vi "Field.vi"(4 "channel 2":T2, 6 "Draw Targets?":T1, 7 "AutoScale":bool=TRUE, 8 "channel for IA State":T3, 10 "Scale mm/pixel":dbl=1.0 format="%#_13g", 11 "channel":T4) -> (2 "Scale Out":dbl, 3 "2D Picture":picture, 5 "AutoScale Out":bool=TRUE)   [LabVIEW 2017]
uses:
  <vilib>/Utility/miscctls.llb/LVBoundsTypeDef.ctl
  <extravilib>/ChannelInstances/Lossy Stream-t'AI Input.ctl'.lvlib
  <extravilib>/ChannelInstances/Lossy Stream-a[.](i32).lvlib
  <extravilib>/ChannelInstances/Lossy Stream-t'SSL Field State.ctl'.lvlib
  Intel/Functions Enum.ctl
  Core/AI Robot.ctl
  Core/AI Ball.ctl
  Core/Field Size.ctl
  Intel/Command Enum.ctl
  Core/AI Judge.ctl
  Core/AI Input.ctl
  <extravilib>/ChannelInstances/Lossy Stream-t'AI Input.ctl'/)Channel.ctl
  <vilib>/Analysis/Matrix/Datatypes/RealMatrix.ctl
  <vilib>/Analysis/Matrix/NI_Matrix.lvlib
  SSL Detection Robot.ctl
  SSL Detection Ball.ctl
  SSL Detection Frame.ctl
  SSL/SSL Field State.ctl
  <extravilib>/ChannelInstances/Lossy Stream-t'SSL Field State.ctl'/)Channel.ctl
  <extravilib>/ChannelInstances/Lossy Stream-a[.](i32)/)Channel.ctl
  Intel/AttackerStates.ctl
  Util/Events/Events.ctl
  DrawTargets.ctl
panel:
  in  "Draw Number":bool=TRUE
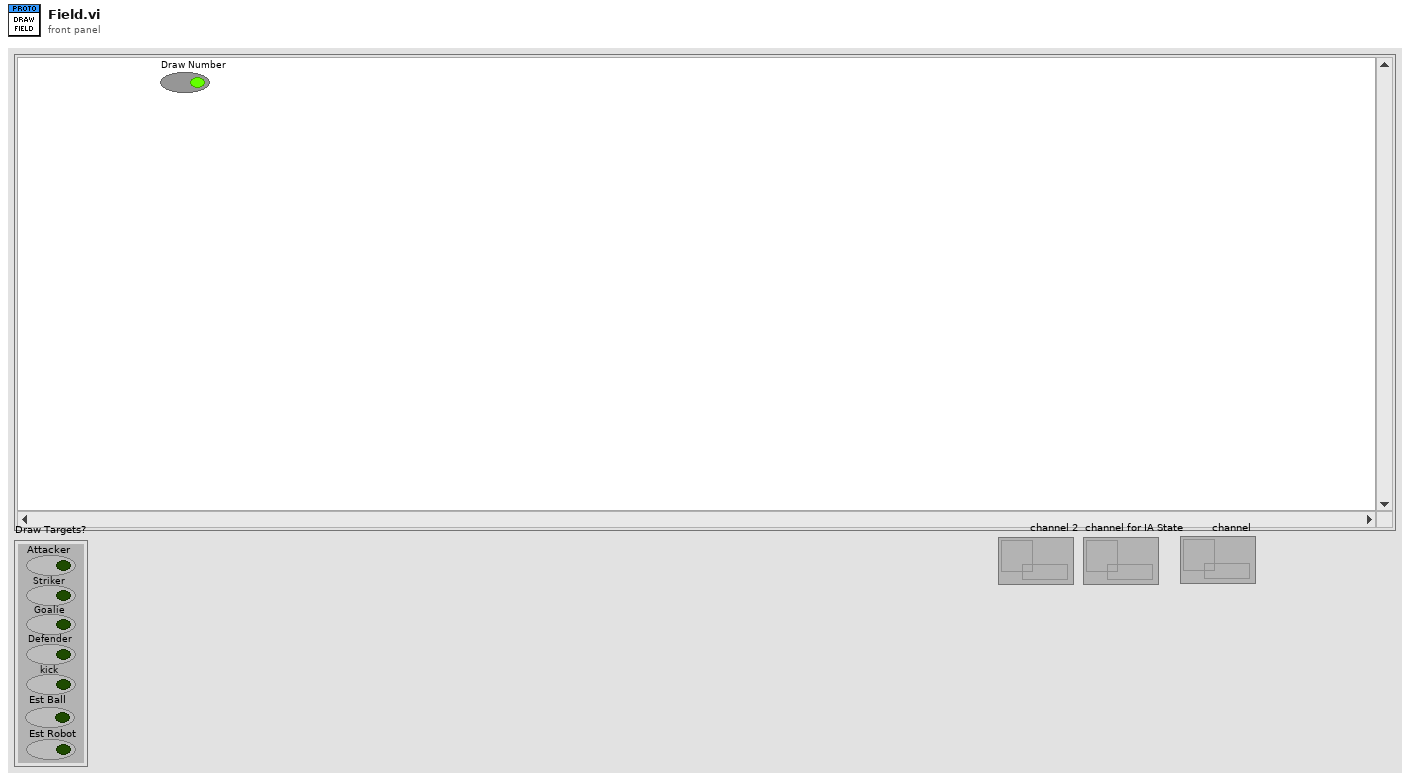
[diagram p1: front panel]
types:
  T1 = typedef "DrawTargets.ctl" = cluster{"Attacker":bool, "Striker":bool, "Goalie":bool, "Defender":bool, "kick":bool, "Est Ball":bool, "Est Robot":bool}
  T2 = typedef "Lossy Stream-a[.](i32).lvlib/)Channel.ctl" = refnum<queue>
  T3 = typedef "Lossy Stream-t'AI Input.ctl'.lvlib/)Channel.ctl" = refnum<queue>
  T4 = typedef "Lossy Stream-t'SSL Field State.ctl'.lvlib/)Channel.ctl" = refnum<queue>
  T5 = typedef "LVBoundsTypeDef.ctl" = cluster{"Width":u32, "Height":u32}
  T6 = typedef "SSL Field State.ctl" = cluster{"Detection Frame Out":T7, "Field Size Out":cluster{"line_width":u32, "field_length":u32, "field_width":u32, "boundary_width":u32, "referee_width":u32, "goal_width":u32, "goal_depth":u32, "goal_wall_width":u32, "center_circle_radius":u32, "defense_radius":u32, "defense_stretch":u32, "free_kick_from_defense_dist":u32, "penalty_spot_from_field_line_dist":u32, "penalty_line_from_spot_dist":u32}, "Received Time Stamp":timestamp}
  T7 = typedef "SSL Detection Frame.ctl" = cluster{"frame_number":u32, "t_capture":dbl, "t_sent":dbl, "camera_id":u32, "robots_yellow":T8[], "robots_blue":T8[], "balls":T10[], "Valid":bool, "Time Stamp":timestamp}
  T8 = typedef "SSL Detection Robot.ctl" = cluster{"x":sgl, "robot_id":u32, "confidence":sgl, "y":sgl, "orientation":sgl, "pixel_x":sgl, "pixel_y":sgl, "height":sgl, "Valid":bool, "Time Stamp":timestamp, "x_k|k":T9, "Pk|k":T9, "Previous Time Stamp":timestamp, "R":T9}
  T9 = typedef "NI_Matrix.lvlib/RealMatrix.ctl" = dbl[][]
  T10 = typedef "SSL Detection Ball.ctl" = cluster{"x":sgl, "area":u32, "confidence":sgl, "y":sgl, "z":sgl, "pixel_x":sgl, "pixel_y":sgl, "Valid":bool, "Time Stamp":timestamp, "x_k|k":T9, "Pk|k":T9, "Id":u32, "Previous Time Stamp":timestamp, "R":T9}
  T11 = typedef "AI Input.ctl" = cluster{"our_robots":T12[], "enemy_robots":T12[], "balls":T15[], "geometry":T16, "IA Judge":T17, "Received Timestamp":timestamp, "Events":T19}
  T12 = typedef "AI Robot.ctl" = cluster{"id":u32, "function":T13, "x":dbl, "y":dbl, "orientation":dbl, "v_tangent":dbl, "v_normal":dbl, "v_ang":dbl, "kick_x":dbl, "kick_z":dbl, "dribble":bool, "Timestamp":timestamp, "dest_x":dbl, "dest_y":dbl, "dest_orientation":dbl, "estimatives":cluster{"est_v_tangent":dbl, "est_v_normal":dbl, "est_vx":dbl, "est_vy":dbl, "Pos Robot Est":dbl[]}, "dest_x_kick":dbl, "dest_y_kick":dbl, "Gap Coord":dbl[], "States":T14}
  T13 = typedef "Functions Enum.ctl" = enum16{"Attacker", "Goalie", "Defender", "Striker", "Goto 0", "Dummy", "Kicker", "ZigZag"}
  T14 = typedef "AttackerStates.ctl" = enum16{"Pass", "GoToTangent", "BallGetting", "GoToKick", ""}
  T15 = typedef "AI Ball.ctl" = cluster{"x":dbl, "y":dbl, "timestamp":timestamp, "Vel_x":dbl, "Vel_y":dbl, "Pos Bola Est":dbl[]}
  T16 = typedef "Field Size.ctl" = cluster{"line_width":u32, "field_length":u32, "field_width":u32, "boundary_width":u32, "referee_width":u32, "goal_width":u32, "goal_depth":u32, "goal_wall_width":u32, "center_circle_radius":u32, "defense_radius":u32, "defense_stretch":u32, "free_kick_from_defense_dist":u32, "penalty_spot_from_field_line_dist":u32, "penalty_line_from_spot_dist":u32}
  T17 = typedef "AI Judge.ctl" = cluster{"stage":string, "command":string, "our_goalie_id":dbl, "enemy_goalie_id":dbl, "command enum":T18, "Time":enum16{"Azul", "Amarelo"}}
  T18 = typedef "Command Enum.ctl" = enum16{"Halt", "Stop", "Force Start", "PKA Normal Start", "Prepare Kickoff Ally", "PKE Normal Start", "Prepare Kickoff Enemy", "Prepare Penalty Ally", "PPA Normal Start", "Prepare Penalty Enemy", "PPE Normal Start", "Direct Free Enemy", "Direct Free Ally", "Indirect Free Enemy", "Indirect Free Ally", "Timeout Enemy", "Timeout Ally", "Goal Enemy", "Goal Ally", "Ball Placement Enemy", "Ball Placement Ally", "Normal Half Time", "Extra Time Break", "Extra Half Time", "None", "Post Game"}
  T19 = typedef "Events.ctl" = cluster{"Touch":bool, "Ball out":bool, "id touch":dbl, "Ball out of \nVision":bool, "Ball inside \nGoalie area":bool, "Robot not responding":bool, "Robots responding status":dbl[], "Enemy Ball \nPossession":bool, "Pass State":bool, "id end of pass":dbl, "Kick":bool, "Id ini Possession":dbl, "Ball Possesion":bool, "Id Possesion":dbl}
  T20 = cluster{"line_width":u32, "field_length":u32, "field_width":u32, "boundary_width":u32, "referee_width":u32, "goal_width":u32, "goal_depth":u32, "goal_wall_width":u32, "center_circle_radius":u32, "defense_radius":u32, "defense_stretch":u32, "free_kick_from_defense_dist":u32, "penalty_spot_from_field_line_dist":u32, "penalty_line_from_spot_dist":u32}
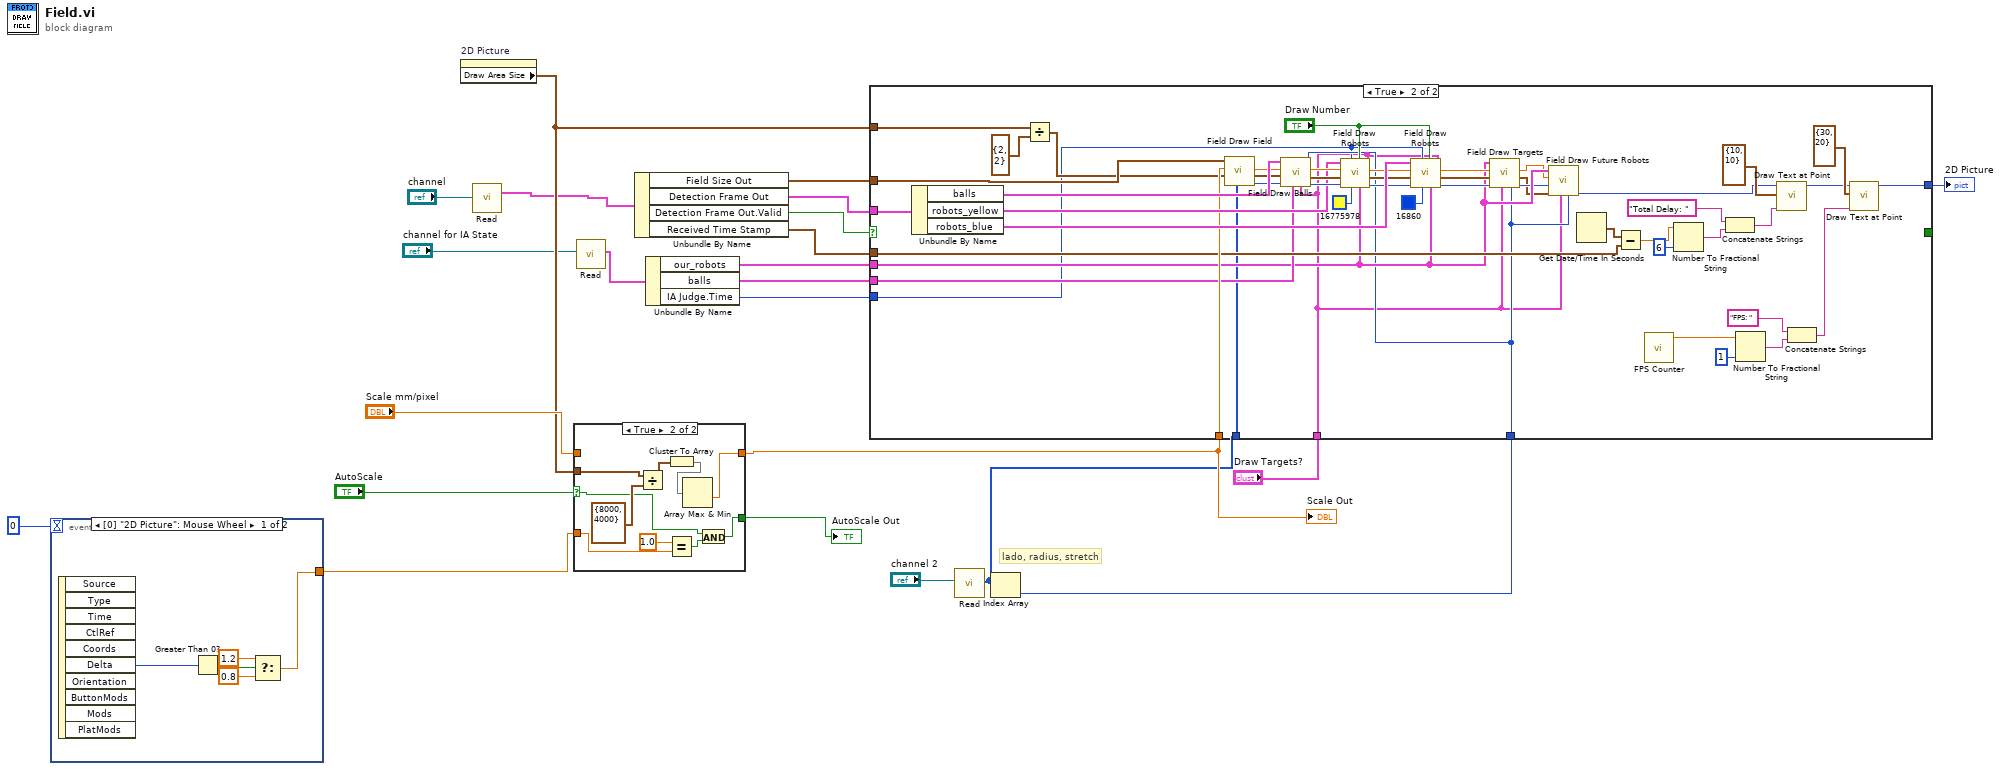
[diagram p0: block diagram]
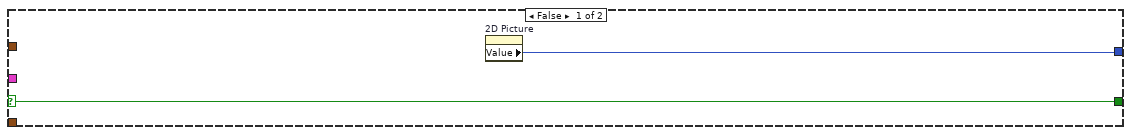
[diagram p2: hidden frame]
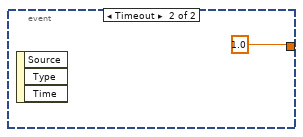
[diagram p3: hidden frame]
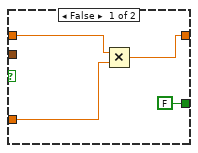
[diagram p4: hidden frame]
diagram:
  # "lado, radius, stretch"
  n1 = event shown="[0] \"2D Picture\": Mouse Wheel" {
    selector: _ -> [_ _]
    dyn-events: _ -> [_ _]
    timeout: 0 -> [_ _]
    tunnel: [w24 1.0] -> w21
    event "2D Picture": Mouse Wheel {
      n2 = event-data() -> ("Delta"=w28:i32)  [unwired: 1 in, 9 out]
      n3 = Greater Than 0?(x=w28) -> (x > 0?=w27:bool)
      n4 = Select(t=1.2, s=w27, f=0.8) -> (s? t:f=w24:dbl)
    }
    event Timeout {
      n5 = event-data() -> ()  [unwired: 1 in, 3 out]
    }
  }
  n6 = property on="2D Picture" class="Pict"() -> ("Draw Area Size"=w20:T5)  [unwired: 2 in, 2 out]
  n7 = call <extravilib>:"Read.vi"("channel"="channel") -> ("element"=w1:T6)  [unwired: 5 in, 5 out]
  n8 = case shown="True" "AutoScale" {
    selector: "AutoScale" -> [_ w35]
    tunnel: "Scale mm/pixel" -> [w33 _]
    tunnel: [w32 w39] -> w15
    tunnel: w20 -> [_ w43]
    tunnel: w21 -> [w31 w38]
    tunnel: [FALSE w36] -> w18
    frame False {
      n9 = Multiply(x=w33, y=w31) -> (x*y=w32:dbl)
    }
    frame True {
      n10 = Divide(x=w43, y=T5 {"Width"=8000, "Height"=4000}) -> (x/y=w41:cluster{"Width":dbl, "Height":dbl})
      n11 = Cluster To Array(cluster=w41) -> (array=w40:dbl[])
      n12 = Equal?(x=1.0, y=w38) -> (x = y?=w34:bool)
      n13 = Array Max & Min(array=w40) -> (min value=w39:dbl)  [unwired: 3 out]
      n14 = And(x=w35, y=w34) -> (x .and. y?=w36:bool)
    }
  }
  "Scale Out" <- w15
  "AutoScale Out" <- w18
  n15 = call <extravilib>:"Read.vi"("channel"="channel for IA State") -> ("element"=w12:T11)  [unwired: 5 in, 5 out]
  n16 = Unbundle By Name(w1) -> ("Field Size Out"=w16:T20, "Detection Frame Out"=w17:T7, "Detection Frame Out.Valid"=w14:bool, "Received Time Stamp"=w13:timestamp)
  n17 = Unbundle By Name(w12) -> ("our_robots"=w11:T12[], "balls"=w6:T15[], "IA Judge.Time"=w3:enum16{"Azul", "Amarelo"})
  n18 = call <extravilib>:"Read.vi"("channel"="channel 2") -> ("element"=w4:i32[])  [unwired: 5 in, 5 out]
  n19 = Index Array(array=w4) -> (element=w9:i32)  [unwired: 1 in]
  n20 = case shown="True" w14 {
    selector: w14 -> [w45 _]
    tunnel: w20 -> [_ w94]
    tunnel: [w44 w67] -> w8
    tunnel: w17 -> [_ w82]
    tunnel: w16 -> [_ w81]
    tunnel: w15 -> [_ w80]
    tunnel: [w45 _] -> _
    tunnel: w13 -> [_ w74]
    tunnel: w11 -> [_ w55]
    tunnel: "Draw Targets?" -> [_ w46]
    tunnel: w9 -> [_ w49]
    tunnel: w6 -> [_ w57]
    tunnel: w4 -> [_ w48]
    tunnel: w3 -> [_ w47]
    frame False {
      n21 = property on="2D Picture" class="Pict"() -> ("Value"=w44:picture)  [unwired: 2 in, 2 out]
    }
    frame True {
      n22 = Unbundle By Name(w82) -> ("balls"=w93:T10[], "robots_yellow"=w89:T8[], "robots_blue"=w88:T8[])
      n23 = Divide(x=w94, y=T5 {"Width"=2, "Height"=2}) -> (x/y=w77:cluster{"Width":dbl, "Height":dbl})
      n24 = call "Field Draw Field.vi"("Lado,radius, stretch"=w48, "Offset"=w77, "Scale"=w80, "Field Size"=w81) -> ("new picture out"=w78:picture, "Offset Out"=w76:cluster{"Width":dbl, "Height":dbl}, "Scale Out"=w79:dbl)  [unwired: 5 in]
      n25 = call "Field Draw Balls.vi"("Lado"=w49, "Draw Targets?"=w46, "balls"=w57, "Picture In"=w78, "Offset"=w76, "Scale"=w79, "Balls"=w93) -> ("Picture Out"=w92:picture, "Offset Out"=w91:cluster{"Width":dbl, "Height":dbl}, "Scale Out"=w90:dbl)  [unwired: 2 in]
      n26 = call "Field Draw Robots.vi"("Draw Targets?"=w46, "our_robots"=w55, "Draw Number"="Draw Number", "color(black)"=u32 16775978, "IA Judge.Time"=w47, "Picture In"=w92, "Offset"=w91, "Scale"=w90, "Detection Robots"=w89) -> ("Picture Out"=w85:picture, "Offset Out"=w86:cluster{"Width":dbl, "Height":dbl}, "Scale Out"=w87:dbl)
      n27 = call "Field Draw Robots.vi"("Draw Targets?"=w46, "our_robots"=w55, "Draw Number"="Draw Number", "color(black)"=u32 16860, "IA Judge.Time"=w47, "Picture In"=w85, "Offset"=w86, "Scale"=w87, "Detection Robots"=w88) -> ("Picture Out"=w59:picture, "Offset Out"=w58:cluster{"Width":dbl, "Height":dbl}, "Scale Out"=w56:dbl)
      n28 = call "Field Draw Targets.vi"("Lado"=w49, "Draw Targets?"=w46, "Picture In"=w59, "Offset"=w58, "Scale"=w56, "our_robots"=w55) -> ("Picture Out"=w54:picture, "Offset Out"=w53:cluster{"Width":dbl, "Height":dbl}, "Scale Out"=w52:dbl)  [unwired: 3 in]
      n29 = call "Field Draw Future Robots.vi"("Lado"=w49, "Draw Targets?"=w46, "Offset"=w53, "Picture In"=w54, "Scale"=w52, "our_robots"=w55) -> ("Picture Out"=w51:picture)  [unwired: 3 in, 2 out]
      n30 = Get Date/Time In Seconds() -> (seconds since 1Jan1904=w73:timestamp)
      n31 = Subtract(x=w73, y=w74) -> (x-y=w72:dbl)
      n32 = call "FPS Counter.vi"() -> ("Numeric"=w63:dbl)  [unwired: 11 in]
      n33 = Number To Fractional String(number=w72, precision (6)=i16 6) -> (F-format string=w70:string)  [unwired: 2 in]
      n34 = Concatenate Strings("Total Delay: " ("text"), w70) -> (w69:string)
      n35 = Number To Fractional String(number=w63, precision (6)=i16 1) -> (F-format string=w65:string)  [unwired: 2 in]
      n36 = call <vilib>:"Draw Text at Point.vi"("text"=w69, "origin"=cluster{"x":i16, "y":i16} {"x"=10, "y"=10}, "picture"=w51) -> ("new picture"=w50:picture)  [unwired: 7 in, 1 out]
      n37 = Concatenate Strings("FPS: " ("text"), w65) -> (w61:string)
      n38 = call <vilib>:"Draw Text at Point.vi"("text"=w61, "origin"=cluster{"x":i16, "y":i16} {"x"=30, "y"=20}, "picture"=w50) -> ("new picture"=w67:picture)  [unwired: 7 in, 1 out]
    }
  }
  "2D Picture" <- w8
